vi "battery_stats.vi"() -> ()   [LabVIEW 2018]
panel:
  out "calculated CRC":u8 format="%02x"
  out "received CRC":u8=19 format="%02x"
  out "CRC matches":bool
  in  "Reset charts":bool
  out "Hours elapsed":dbl
  out "WH":dbl format="%_4p"
  out "Temperature":waveform(u8)[](graph)
  out "time since":dbl caption="seconds since\nvalid packet" format="%.3g"
  out "32-bit UINT seconds since 1900":u32=4294967295 format="%.0x"
  out "time stamp from 32bit binary":timestamp
  out "time stamp from string":timestamp
  out "Amps/Watts":waveform(sgl)[](graph)
  out "Volts":waveform(sgl)[](graph)
  in  "port":u16=5606
  out "error out":errorcluster
  in  "stop":bool
  out "actual port used":u16
  out "incoming data":string
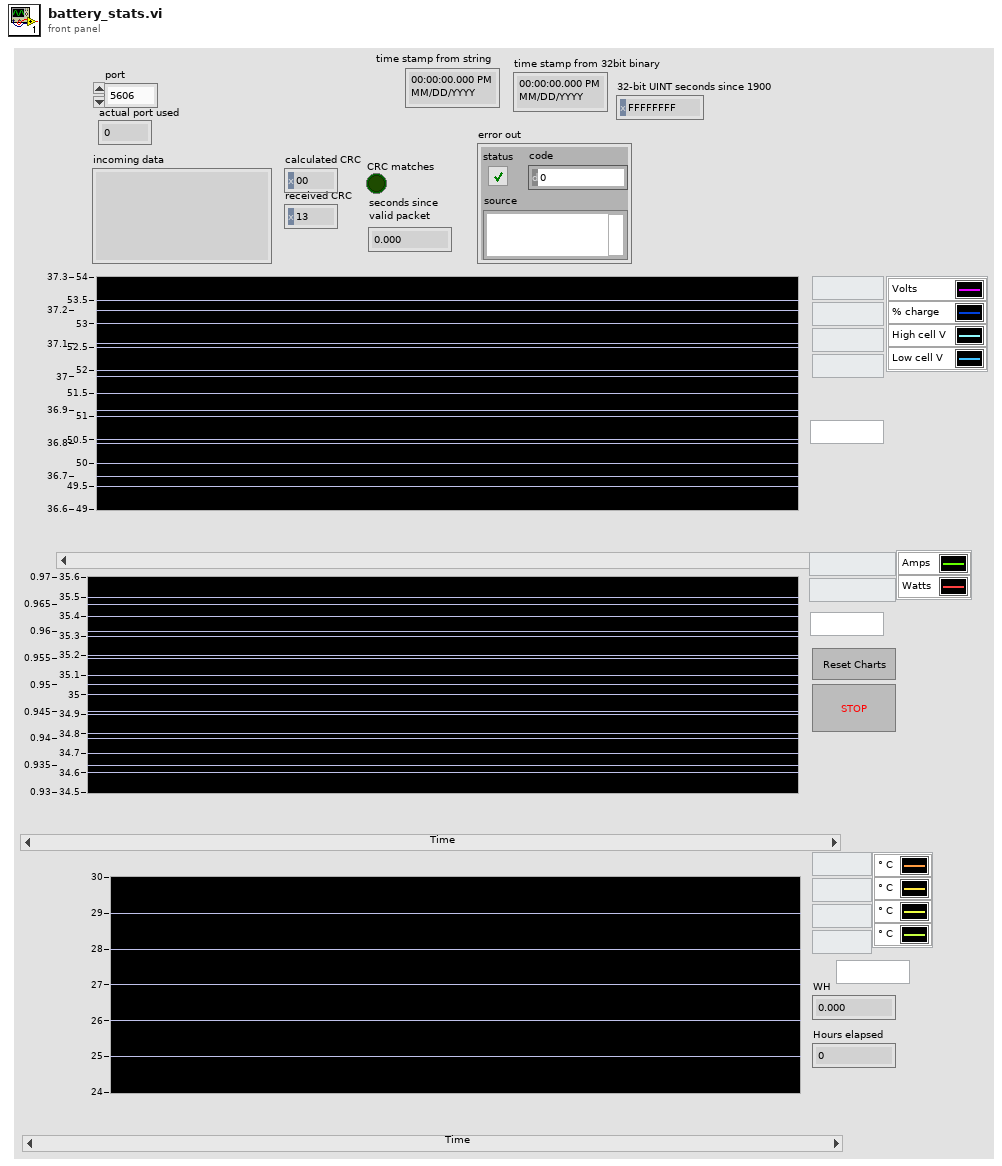
[diagram p1: front panel]
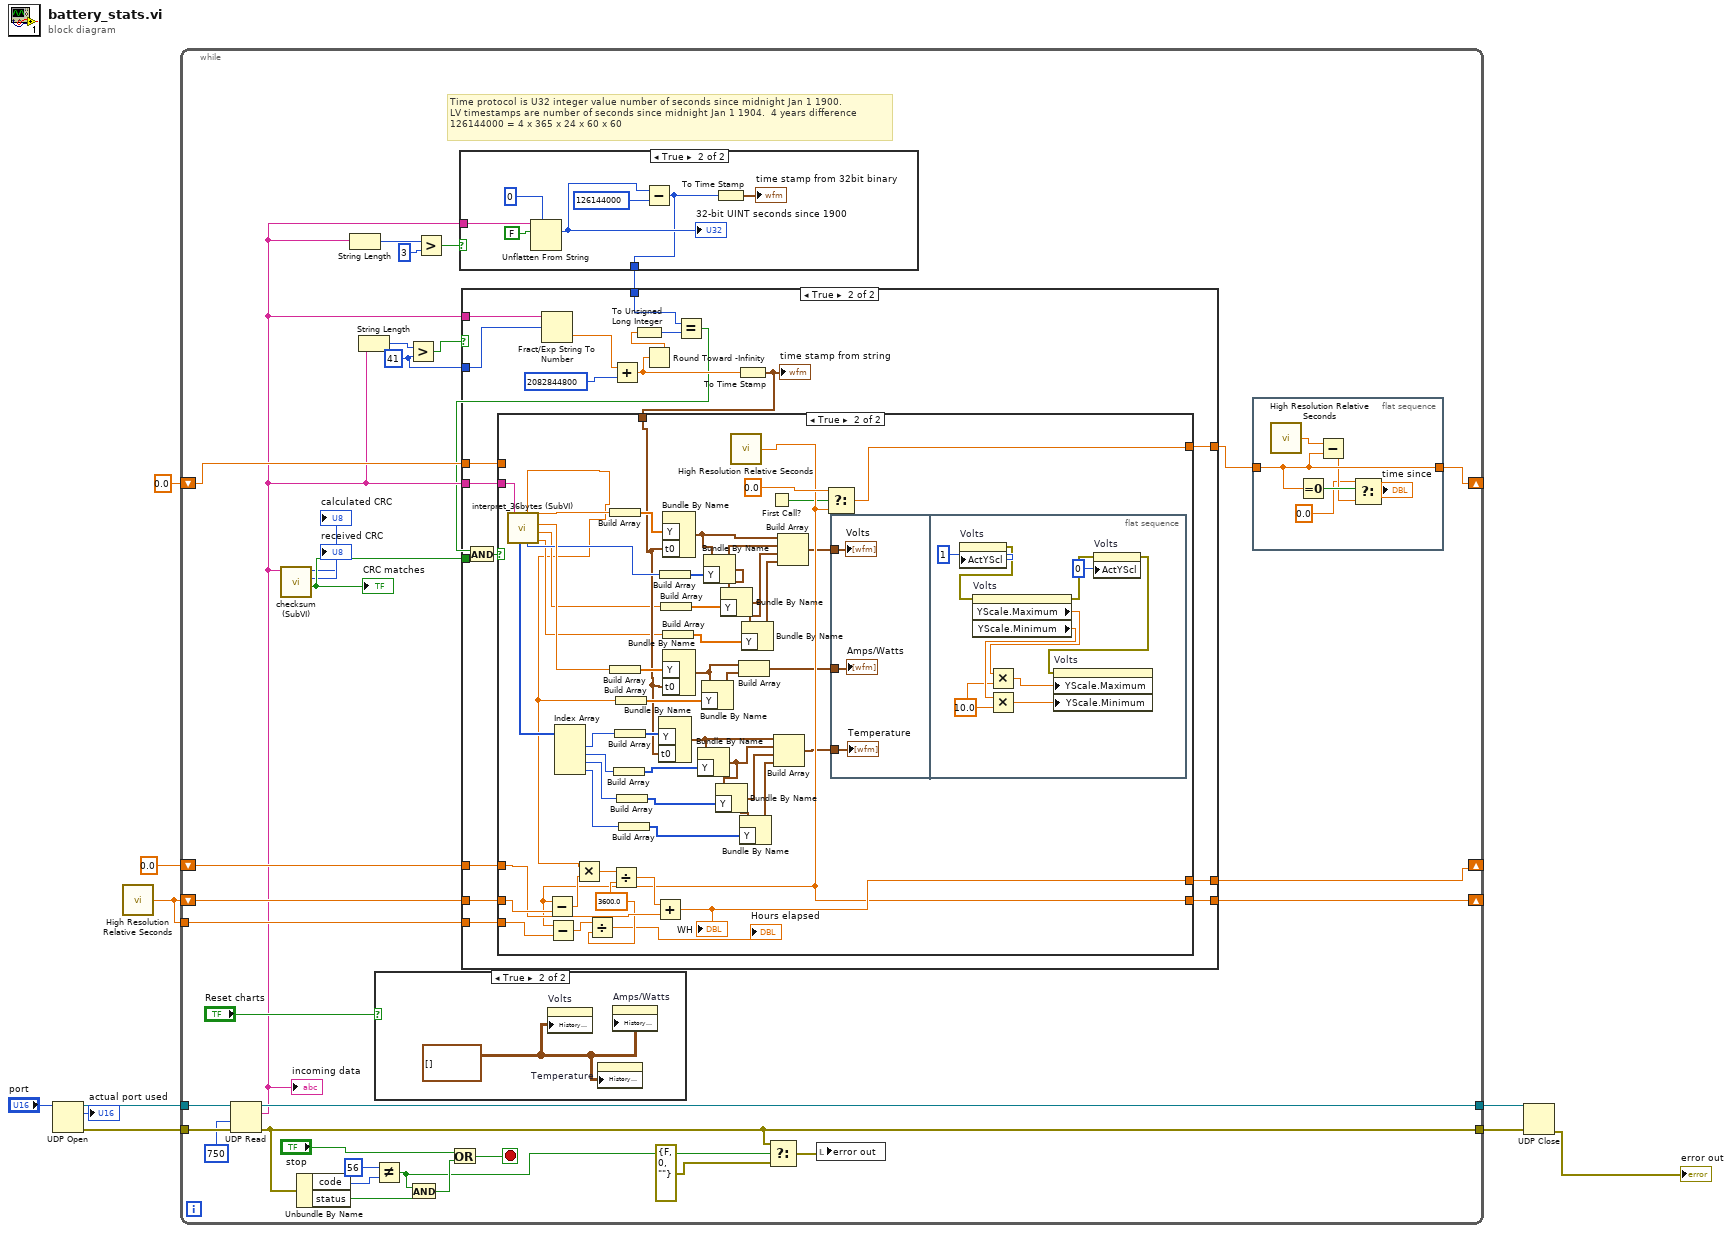
[diagram p0: block diagram]
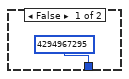
[diagram p5: hidden frame]
diagram:
  n1 = UDP Open(11:"port") -> (port=w9:refnum<k16>, 0:w8:errorcluster, 2:→"actual port used":u16)  [unwired: 4 in]
  n2 = call <vilib>:"High Resolution Relative Seconds.vi"() -> ("relative seconds"=w1:dbl)
  n3 = while {
    tunnel: w9 -> [w44]
    tunnel: [w26] -> w6
    tunnel: [w34] -> w5
    tunnel: w8 -> [w43]
    shift-right: [w22] -> _
    shift-left: 0.0 ("relative seconds") -> [w24]
    shift-right: [w19] -> _
    shift-left: sgl 0.0 ("relative seconds") -> [w20]
    shift-right: [w17] -> _
    shift-left: w1 -> [w18]
    tunnel: w1 -> [w16]
    stop <- w42 stop-if-true
    w36 = 41 ("y")
    # "Time protocol is U32 integer value number of seconds since midnight Jan 1 1900.\nLV timestamps are number of seconds since midnight Jan 1 1904.  4 years difference\n126144000 = 4 x 365 x 24 x 60 x 60"
    n4 = UDP Read(connection ID=w44, timeout ms (25000)=750, 8:w43) -> (data out=w14:string, error out=w26:errorcluster, 3:w34:refnum<k16>)  [unwired: 1 in, 2 out]
    "incoming data" <- w14
    n5 = call "checksum (SubVI).vi"("incoming data"=w14) -> ("CRC matches"=w13:bool, "received CRC"=→"received CRC":u8, "calculated CRC"=→"calculated CRC":u8)  [unwired: 8 in]
    "CRC matches" <- w13
    n6 = Unbundle By Name(w26) -> ("code"=w31:i32, "status"=w28:bool)
    n7 = String Length(string=w14) -> (length=w41:i32)
    n8 = String Length(string=w14) -> (length=w38:i32)
    n9 = Not Equal?(x=56, y=w31) -> (x != y?=w27:bool)
    n10 = case shown="True" "Reset charts" {
      frame False {
      }
      frame True {
        w45 = waveform(sgl)[][] [] ("History Data")
        n11 = property on="Volts" class="WFChart (strict)"("History Data"=w45) -> ()  [unwired: 2 in, 2 out]
        n12 = property on="Temperature" class="WFChart (strict)"("History Data"=w45) -> ()  [unwired: 2 in, 2 out]
        n13 = property on="Amps/Watts" class="WFChart (strict)"("History Data"=w45) -> ()  [unwired: 2 in, 2 out]
      }
    }
    n14 = Greater?(x=w38, y=w36) -> (0:w37:bool)
    n15 = And(x=w27, y=w28) -> (x .and. y?=w29:bool)
    n16 = Greater?(x=w41, y=3) -> (0:w39:bool)
    n17 = Or(x="stop", y=w29) -> (x .or. y?=w42:bool)
    n18 = case shown="True" w39 {
      tunnel: w14 -> [_ w148]
      tunnel: [u32 4294967295 w142] -> w35
      frame False {
      }
      frame True {
        n19 = Unflatten From String(type=u32 0, binary string=w148, data includes array or string size? (T)=FALSE) -> (value=w143:u32)  [unwired: 2 in, 2 out]
        "32-bit UINT seconds since 1900" <- w143
        n20 = Subtract(x=w143, y=u32 126144000) -> (x-y=w142:u32)
        n21 = To Time Stamp(1:w142) -> (0:→"time stamp from 32bit binary":timestamp)
      }
    }
    n22 = case shown="True" w37 {
      tunnel: w14 -> [_ w74]
      tunnel: w36 -> [_ w73]
      tunnel: w35 -> [_ w69]
      tunnel: w14 -> [_ w68]
      tunnel: w24 -> [w54 w64]
      tunnel: [w54 w63] -> w23
      tunnel: w20 -> [w53 w62]
      tunnel: [w53 w61] -> w19
      tunnel: w18 -> [w52 w60]
      tunnel: [w52 w59] -> w17
      tunnel: w16 -> [_ w58]
      tunnel: w13 -> [_ w56]
      frame False {
      }
      frame True {
        n23 = Fract/Exp String To Number(string=w74, offset=w73) -> (number=w71:dbl)  [unwired: 2 in, 1 out]
        n24 = Add(x=w71, y=u32 2082844800 ("x")) -> (x+y=w66:dbl)
        n25 = Round Toward -Infinity(1:w66) -> (0:w65:dbl)
        n26 = To Unsigned Long Integer(number=w65) -> (unsigned 32bit integer=w70:u32)
        n27 = Equal?(x=w69, y=w70) -> (x = y?=w57:bool)
        n28 = And(x=w57, y=w56) -> (x .and. y?=w55:bool)
        n29 = To Time Stamp(1:w66) -> (0:w67:timestamp)
        "time stamp from string" <- w67
        n30 = case shown="True" w55 {
          tunnel: w68 -> [_ w125]
          tunnel: w67 -> [_ w86]
          tunnel: w64 -> [w77 _]
          tunnel: [w77 w123] -> w63
          tunnel: w62 -> [w76 w116]
          tunnel: [w76 w115] -> w61
          tunnel: w60 -> [w75 w119]
          tunnel: [w75 w110] -> w59
          tunnel: w58 -> [_ w109]
          frame False {
          }
          frame True {
            w113 = 3600.0 ("y")
            n31 = call "interpret_36bytes (SubVI).vi"("data in"=w125) -> ("low cell, V"=w80:sgl, "high cell, V"=w79:sgl, "Amps"=w121:sgl, "Volts"=w120:sgl, "% charged"=w103:u8, "Watts"=w78:sgl, "temperature °C"=w95:u8[])  [unwired: 4 in]
            n32 = Index Array(array=w95) -> (element #1=w94:u8, element #2=w93:u8, element #3=w92:u8, element #4=w91:u8)  [unwired: 4 in]
            n33 = Build Array(w120) -> (w126:sgl[])
            n34 = Build Array(w121) -> (w127:sgl[])
            n35 = Build Array(w93) -> (w89:u8[])
            n36 = Build Array(w94) -> (w90:u8[])
            n37 = Build Array(w78) -> (w122:sgl[])
            n38 = Build Array(w92) -> (w88:u8[])
            n39 = Build Array(w91) -> (w87:u8[])
            n40 = Bundle By Name("Y"=w90, "t0"=w86) -> (w100:waveform(u8))  [unwired: 1 in]
            n41 = Build Array(w103) -> (w104:u8[])
            n42 = Build Array(w79) -> (w81:sgl[])
            n43 = Bundle By Name("Y"=w126, "t0"=w86) -> (w102:waveform(sgl))  [unwired: 1 in]
            n44 = Build Array(w80) -> (w82:sgl[])
            n45 = Bundle By Name("Y"=w127, "t0"=w86) -> (w108:waveform(sgl))  [unwired: 1 in]
            n46 = Bundle By Name(cluster=w100, "Y"=w89) -> (w99:waveform(u8))
            n47 = Bundle By Name(cluster=w108, "Y"=w122) -> (w107:waveform(sgl))
            n48 = Bundle By Name(cluster=w102, "Y"=w104) -> (w85:waveform(sgl))
            n49 = Bundle By Name(cluster=w99, "Y"=w88) -> (w98:waveform(u8))
            n50 = Bundle By Name(cluster=w85, "Y"=w81) -> (w84:waveform(sgl))
            n51 = call <vilib>:"High Resolution Relative Seconds.vi"() -> ("relative seconds"=w110:dbl)
            n52 = Subtract(x=w110, y=w119) -> (x-y=w114:dbl)
            n53 = Subtract(x=w110, y=w109) -> (x-y=w111:dbl)
            n54 = Multiply(x=w78, y=w114) -> (x*y=w118:dbl)
            n55 = Divide(x=w111, y=w113) -> (x/y=→"Hours elapsed":dbl)
            n56 = Divide(x=w118, y=w113) -> (x/y=w117:dbl)
            n57 = Add(x=w117, y=w116) -> (x+y=w115:dbl)
            "WH" <- w115
            n58 = Build Array(w108, w107) -> (w106:waveform(sgl)[])
            n59 = Bundle By Name(cluster=w98, "Y"=w87) -> (w97:waveform(u8))
            n60 = Bundle By Name(cluster=w84, "Y"=w82) -> (w83:waveform(sgl))
            n61 = First Call?() -> (First Call?: T/F=w105:bool)
            n62 = Build Array(w100, w99, w98, w97) -> (w96:waveform(u8)[])
            n63 = Build Array(w102, w85, w84, w83) -> (w101:waveform(sgl)[])
            n64 = Select(t=0.0, s=w105, f=w110) -> (s? t:f=w123:dbl)
            n65 = flat-sequence {
              tunnel: w106 -> [w130]
              tunnel: w101 -> [w129]
              tunnel: w96 -> [w128]
              frame #0 {
                "Volts" <- w129
                "Amps/Watts" <- w130
                "Temperature" <- w128
              }
              frame #1 {
                w131 = 10.0 ("y")
                n66 = property on="Volts" class="WFChart (strict)"("ActYScl"=1 ("Active Y Scale")) -> (error out=w139:errorcluster)  [unwired: 2 in, 1 out]
                n67 = property on="Volts" class="WFChart (strict)"(error in=w139) -> (error out=w138:errorcluster, "YScale.Maximum"=w135:dbl, "YScale.Minimum"=w133:dbl)  [unwired: 1 in, 1 out]
                n68 = Multiply(x=w135, y=w131) -> (x*y=w134:dbl)
                n69 = Multiply(x=w133, y=w131) -> (x*y=w132:dbl)
                n70 = property on="Volts" class="WFChart (strict)"(error in=w138, "ActYScl"=0 ("Active Y Scale")) -> (error out=w136:errorcluster)  [unwired: 1 in, 1 out]
                n71 = property on="Volts" class="WFChart (strict)"(error in=w136, "YScale.Maximum"=w134, "YScale.Minimum"=w132) -> ()  [unwired: 1 in, 2 out]
              }
            }
          }
        }
      }
    }
    n72 = Select(t=w26, s=w27, f=errorcluster {"status"=FALSE, "code"=0, "source"=""} ("error in (no error)")) -> (s? t:f=w25:errorcluster)
    n73 = local write "error out"(w25) -> ()
    n74 = flat-sequence {
      tunnel: [w49] -> w22
      tunnel: w23 -> [w49]
      frame #0 {
        n75 = call <vilib>:"High Resolution Relative Seconds.vi"() -> ("relative seconds"=w51:dbl)
        n76 = Equal To 0?(x=w49) -> (x = 0?=w50:bool)
        n77 = Subtract(x=w51, y=w49) -> (x-y=w48:dbl)
        n78 = Select(t=0.0, s=w50, f=w48) -> (s? t:f=→"time since":dbl)
      }
    }
  }
  n79 = UDP Close(connection ID=w5, 8:w6) -> (error out=→"error out":errorcluster)  [unwired: 1 out]
